vi "Chrg_Dschrg.vi"() -> ()   [LabVIEW 2020]
uses:
  <instrlib>/NH Research Regenerative Test Series/Public/Data/Read (Ave Current).vi
  <instrlib>/NH Research Regenerative Test Series/Public/Data/Low Level/Fetch (Ave Voltage).vi
  <instrlib>/NH Research Regenerative Test Series/NH Research Regenerative Test Series.lvlib
  <instrlib>/IT-M3400/IT-M3400.lvlib
panel:
  in  "Battery Type":enum16{"30Q", "40T"}(ring)
  in  "PS type":enum16{"NHR", "ITECH"}(ring)
  in  "#DAQ outputs (1-13)":i32
  out "Read Ave Current (A)":dbl
  out "Read Ave Voltage (V)":dbl
  in  "Charge/discharge":enum8{"Charge", "Discharge"}(ring)
  out "NHR error out":errorcluster
  out "VISA resource name out":refnum<visa-resource-name>
  out "data task error out":errorcluster
  out "data task out":refnum<k21>
  in  "DischargeCyclePath":path=path "C:/Users/ga11/Desktop/VI/results/3PtestCharge.lvm" caption="Filename"
  in  "Data Task in":refnum<k21>
  in  "data task error in":errorcluster
  in  "PS error in":errorcluster caption="NHR error in (no error)"
  in  "PS VISA in":refnum<visa-resource-name>
  in  "Current Setpoint":dbl format="%#.6g"
  in  "Current Cutoff":dbl
  in  "Charge/Discharge Voltage Setpoint":dbl format="%#.6g"
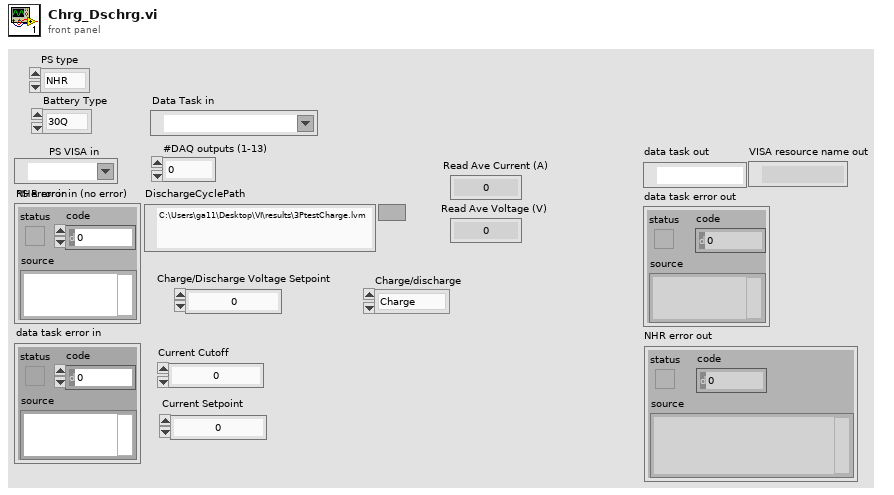
[diagram p1: front panel]
types:
  T1 = cluster{"Voltage Enabled":bool, "Current Enabled":bool, "Power Enabled":bool, "Resistance Enabled":bool}
  T2 = cluster{"Baud Rate":u32, "Parity":u16, "Data Bits":u16, "Stop Bits":u16, "Flow Control":u16}
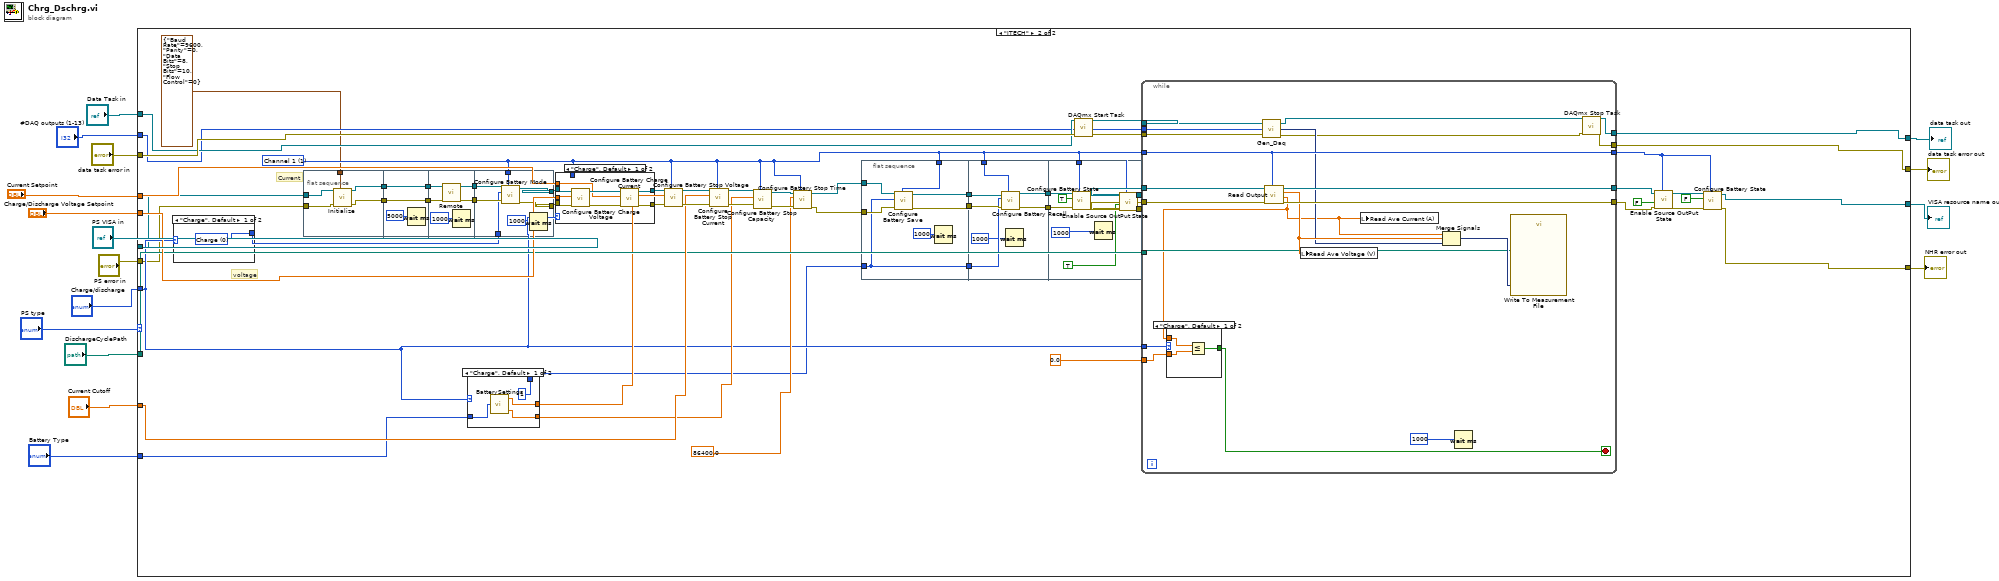
[diagram p0: block diagram]
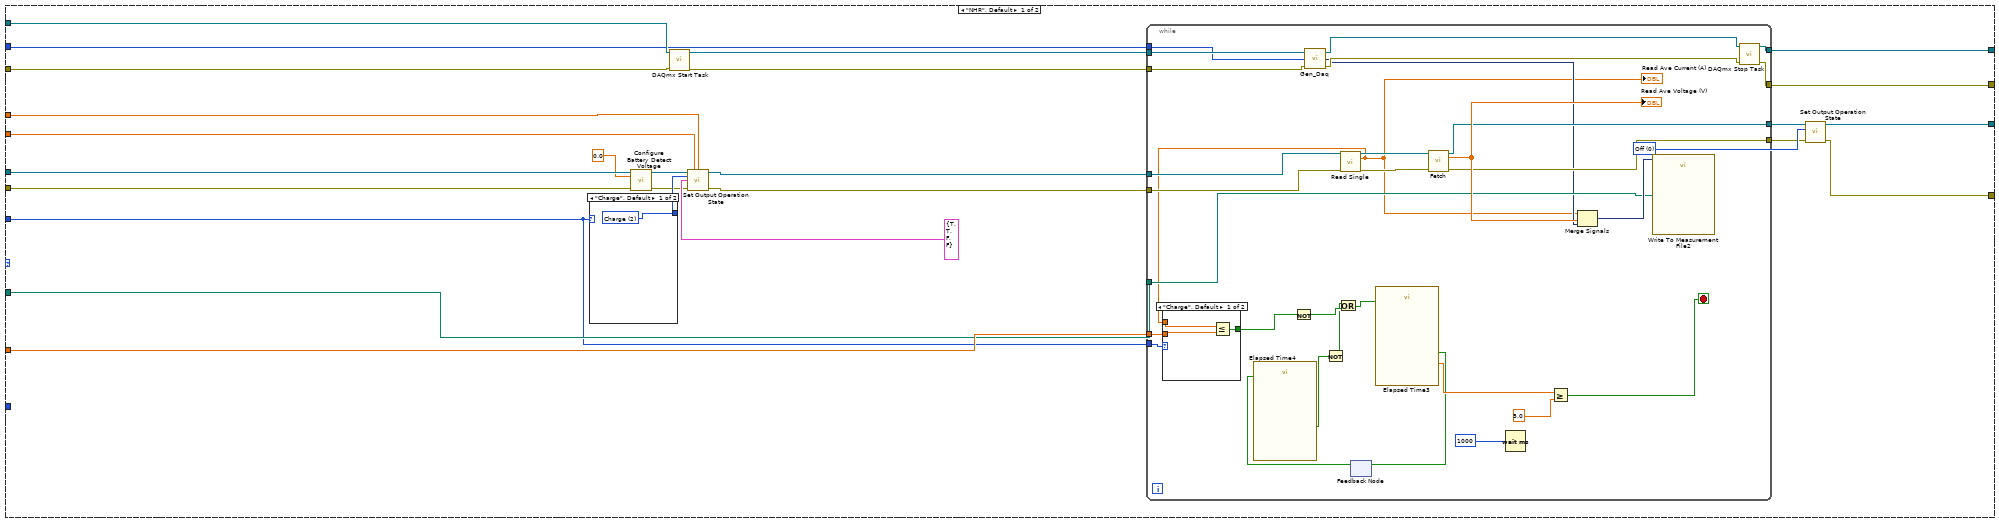
[diagram p2: hidden frame]
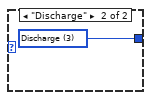
[diagram p3: hidden frame]
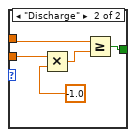
[diagram p4: hidden frame]
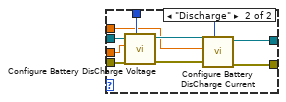
[diagram p5: hidden frame]
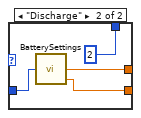
[diagram p6: hidden frame]
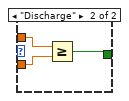
[diagram p7: hidden frame]
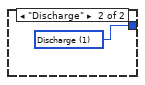
[diagram p8: hidden frame]
diagram:
  n1 = case shown="\"ITECH\"" "PS type" {
    tunnel: "Charge/Discharge Voltage Setpoint" -> [w42 w119]
    tunnel: "Current Setpoint" -> [w17 w112]
    tunnel: "Current Cutoff" -> [w39 w114]
    tunnel: "DischargeCyclePath" -> [w36 w113]
    tunnel: "Data Task in" -> [w33 w120]
    tunnel: "data task error in" -> [w32 w121]
    tunnel: "PS VISA in" -> [w28 w85]
    tunnel: "PS error in" -> [w27 w84]
    tunnel: [w25 w118] -> w8
    tunnel: [w24 w116] -> w7
    tunnel: [w23 w117] -> w6
    tunnel: [w22 w115] -> w5
    tunnel: "Charge/discharge" -> [w18 w106]
    tunnel: "#DAQ outputs (1-13)" -> [w19 w92]
    tunnel: "Battery Type" -> [_ w111]
    frame "NHR", Default {
      w31 = 0 items=["Off", "Standby", "Charge", "Discharge", "Battery"] ("Mode (0: Off)")
      n2 = case shown="\"Charge\", Default" w18 {
        tunnel: [w43 w44] -> w37
        frame "Charge", Default {
          w43 = 2 items=["Off", "Standby", "Charge", "Discharge", "Battery"] ("Mode (0: Off)")
        }
        frame "Discharge" {
          w44 = 3 items=["Off", "Standby", "Charge", "Discharge", "Battery"] ("Mode (0: Off)")
        }
      }
      n3 = call <instrlib>:"Configure Battery Detect Voltage.vi"("VISA resource name"=w28, "Battery Detect Voltage (0V)"=0.0, "error in (no error)"=w27) -> ("VISA resource name out"=w30:refnum<visa-resource-name>, "error out"=w29:errorcluster)  [unwired: 11 in]
      n4 = call <vilib>:"DAQmx Start Task.vi"("task/channels in"=w33, "error in"=w32) -> ("task out"=w35:refnum<k21>, "error out"=w34:errorcluster)  [unwired: 12 in]
      n5 = call <vilib>:"Set Output Operation State.vi"("VISA resource name"=w30, "Voltage Setpoint (0 V)"=w42, "Current Setpoint (0 A)"=w17, "Mode (0: Off)"=w37, "Enable"=T1 {"Voltage Enabled"=TRUE, "Current Enabled"=TRUE, "Power Enabled"=FALSE, "Resistance Enabled"=FALSE}, "error in (no error)"=w29) -> ("VISA resource name out"=w41:refnum<visa-resource-name>, "error out"=w40:errorcluster)  [unwired: 8 in]
      n6 = while {
        tunnel: w41 -> [w73]
        tunnel: w40 -> [w72]
        tunnel: w39 -> [w48]
        tunnel: w34 -> [w53]
        tunnel: w35 -> [w54]
        tunnel: w36 -> [w59]
        tunnel: [w58] -> w25
        tunnel: [w57] -> w23
        tunnel: [w56] -> w21
        tunnel: [w55] -> w20
        tunnel: w19 -> [w52]
        tunnel: w18 -> [w47]
        stop <- w62 stop-if-true
        n7 = call "Gen_Daq.vi"("error in"=w53, "#DAQ outputs (1-13)"=w52, "task/channels in"=w54) -> ("error out"=w50:errorcluster, "DaQ_output"=w49:dynamicdata, "task out"=w51:refnum<k21>)
        n8 = call-poly <instrlib>:"Read Single.vi"("VISA resource name"=w73, "error in (no error)"=w72) -> ("VISA resource name out"=w74:refnum<visa-resource-name>, "Ave Current (A)"=w46:dbl, "error out"=w75:errorcluster)  [unwired: 11 in]
        "Read Ave Current (A)" <- w46
        n9 = case shown="\"Charge\", Default" w47 {
          tunnel: w48 -> [w77 w82]
          tunnel: w46 -> [w78 w80]
          tunnel: [w76 w79] -> w45
          frame "Charge", Default {
            n10 = Less Or Equal?(x=w78, y=w77) -> (x <= y?=w76:bool)
          }
          frame "Discharge" {
            n11 = Multiply(x=w82, y=-1.0) -> (x*y=w81:dbl)
            n12 = Greater Or Equal?(x=w80, y=w81) -> (x >= y?=w79:bool)
          }
        }
        n13 = Not(x=w45) -> (.not. x?=w68:bool)
        n14 = feedback #1() -> (w60:bool)  [unwired: 1 in]
        n15 = call "Elapsed Time4"("Reset"=w60) -> ("Time has Elapsed"=w67:bool)  [unwired: 11 in, 7 out]
        n16 = Not(x=w67) -> (.not. x?=w66:bool)
        n17 = Or(x=w66, y=w68) -> (x .or. y?=w65:bool)
        n18 = call "Elapsed Time3"("Reset"=w65) -> ("Elapsed Time (s)"=w64:dbl, "Time has Elapsed"=w61:bool)  [unwired: 11 in, 6 out]
        n19 = feedback-in #1(w61) -> ()
        n20 = call-poly <instrlib>:"Fetch.vi"("VISA resource name"=w74, "error in (no error)"=w75) -> ("VISA resource name out"=w56:refnum<visa-resource-name>, "Ave Voltage (V)"=w70:dbl, "error out"=w55:errorcluster)  [unwired: 11 in]
        "Read Ave Voltage (V)" <- w70
        n21 = Wait (ms)(milliseconds to wait=1000) -> ()  [unwired: 1 out]
        n22 = Greater Or Equal?(x=w64, y=5.0) -> (x >= y?=w62:bool)
        n23 = Merge Signals "Merge Signals"(w46, w70, w49) -> (w71:dynamicdata)
        n24 = call "Write To Measurement File2"("Signals"=w71, "Filename"=w59) -> ()  [unwired: 15 in, 3 out]
        n25 = call <vilib>:"DAQmx Stop Task.vi"("task/channels in"=w51, "error in"=w50) -> ("task out"=w58:refnum<k21>, "error out"=w57:errorcluster)  [unwired: 12 in]
      }
      n26 = call <vilib>:"Set Output Operation State.vi"("VISA resource name"=w21, "Mode (0: Off)"=w31, "error in (no error)"=w20) -> ("VISA resource name out"=w24:refnum<visa-resource-name>, "error out"=w22:errorcluster)  [unwired: 11 in]
    }
    frame "ITECH" {
      w91 = 1 items=["Channel 1"=1, "Channel 2"=2, "Channel 3"=3, "Channel 4"=4, "Channel 5"=5, "Channel 6"=6, "Channel 7"=7, "Channel 8"=8, "Channel 8"=9, "Channel 10"=10, "Channel 11"=11, "Channel 12"=12, "Channel 13"=13, "Channel 14"=14, "Channel 15"=15, "Channel 16"=16] ("Channel")
      # "voltage"
      # "Current"
      n27 = case shown="\"Charge\", Default" w106 {
        tunnel: [w237 w238] -> w95
        frame "Charge", Default {
          w237 = u8 0 items=["Charge", "Discharge"] ("Battery Mode")
        }
        frame "Discharge" {
          w238 = u8 1 items=["Charge", "Discharge"] ("Battery Mode")
        }
      }
      n28 = flat-sequence {
        tunnel: [w141] -> w89
        tunnel: [w142] -> w87
        tunnel: T2 {"Baud Rate"=9600, "Parity"=0, "Data Bits"=8, "Stop Bits"=10, "Flow Control"=0} ("Serial Configuration") -> [w145]
        tunnel: w84 -> [w144]
        tunnel: w85 -> [w143]
        tunnel: w89 -> [w148]
        tunnel: [w148] -> w88
        tunnel: w87 -> [w147]
        tunnel: [w147] -> w86
        tunnel: [w153] -> w97
        tunnel: [w152] -> w96
        tunnel: w88 -> [w151]
        tunnel: w86 -> [w150]
        tunnel: w97 -> [w157]
        tunnel: w96 -> [w159]
        tunnel: w91 -> [w160]
        tunnel: w95 -> [w158]
        tunnel: [w156] -> w94
        tunnel: [w155] -> w93
        frame #0 {
          n29 = call <instrlib>:"Initialize.vi"("Serial Configuration"=w145, "error in"=w144, "VISA resource name"=w143) -> ("error out"=w142:errorcluster, "VISA resource name out"=w141:refnum<visa-resource-name>)  [unwired: 7 in]
        }
        frame #1 {
          n30 = Wait (ms)(milliseconds to wait=5000) -> ()  [unwired: 1 out]
        }
        frame #2 {
          n31 = call <instrlib>:"Remote.vi"("error in"=w150, "VISA resource name"=w151) -> ("error out"=w152:errorcluster, "VISA resource name out"=w153:refnum<visa-resource-name>)  [unwired: 8 in]
          n32 = Wait (ms)(milliseconds to wait=1000) -> ()  [unwired: 1 out]
        }
        frame #3 {
          n33 = call <instrlib>:"Configure Battery Mode.vi"("Channel"=w160, "error in"=w159, "Battery Mode"=w158, "VISA resource name"=w157) -> ("error out"=w156:errorcluster, "VISA resource name out"=w155:refnum<visa-resource-name>)  [unwired: 6 in]
          n34 = Wait (ms)(milliseconds to wait=1000) -> ()  [unwired: 1 out]
        }
      }
      n35 = case shown="\"Charge\", Default" w106 {
        tunnel: w111 -> [w205 w209]
        tunnel: [w204 w208] -> w110
        tunnel: [w203 w207] -> w109
        tunnel: [u8 1 ("File") u8 2 ("File")] -> w103
        frame "Charge", Default {
          n36 = call "BatterySettings.vi"("Battery Type"=w205) -> ("RatedCapacity (Ah)"=w203:dbl, "Max Voltage (V)"=w204:dbl)  [unwired: 2 in, 1 out]
        }
        frame "Discharge" {
          n37 = call "BatterySettings.vi"("Battery Type"=w209) -> ("RatedCapacity (Ah)"=w207:dbl, "Min Voltage (V)"=w208:dbl)  [unwired: 2 in, 1 out]
        }
      }
      n38 = case shown="\"Charge\", Default" w106 {
        tunnel: w93 -> [w192 w201]
        tunnel: w94 -> [w191 w200]
        tunnel: [w186 w197] -> w130
        tunnel: [w185 w196] -> w129
        tunnel: w91 -> [_ w195]
        tunnel: w119 -> [w188 w194]
        tunnel: w112 -> [w187 w193]
        frame "Charge", Default {
          n39 = call <instrlib>:"Configure Battery Charge Voltage.vi"("error in"=w191, "Charge Voltage(V)"=w188, "VISA resource name"=w192) -> ("error out"=w189:errorcluster, "VISA resource name out"=w190:refnum<visa-resource-name>)  [unwired: 6 in]
          n40 = call <instrlib>:"Configure Battery Charge Current.vi"("error in"=w189, "Charge Current(A)"=w187, "VISA resource name"=w190) -> ("error out"=w185:errorcluster, "VISA resource name out"=w186:refnum<visa-resource-name>)  [unwired: 7 in]
        }
        frame "Discharge" {
          n41 = call <instrlib>:"Configure Battery DisCharge Voltage.vi"("Channel"=w195, "error in"=w200, "Discharge Voltage(V)"=w194, "VISA resource name"=w201) -> ("error out"=w198:errorcluster, "VISA resource name out"=w199:refnum<visa-resource-name>)  [unwired: 6 in]
          n42 = call <instrlib>:"Configure Battery DisCharge Current.vi"("Channel"=w195, "error in"=w198, "Discharge Current(A)"=w193, "VISA resource name"=w199) -> ("error out"=w196:errorcluster, "VISA resource name out"=w197:refnum<visa-resource-name>)  [unwired: 6 in]
        }
      }
      n43 = call <instrlib>:"Configure Battery Stop Voltage.vi"("Channel"=w91, "error in"=w129, "Stop Voltage(V)"=w110, "VISA resource name"=w130) -> ("error out"=w139:errorcluster, "VISA resource name out"=w140:refnum<visa-resource-name>)  [unwired: 6 in]
      n44 = call <instrlib>:"Configure Battery Stop Current.vi"("Channel"=w91, "error in"=w139, "Stop Current(A)"=w114, "VISA resource name"=w140) -> ("error out"=w137:errorcluster, "VISA resource name out"=w138:refnum<visa-resource-name>)  [unwired: 6 in]
      n45 = call <instrlib>:"Configure Battery Stop Capacity.vi"("Channel"=w91, "error in"=w137, "Stop Capacity(Ah)"=w109, "VISA resource name"=w138) -> ("error out"=w135:errorcluster, "VISA resource name out"=w136:refnum<visa-resource-name>)  [unwired: 6 in]
      n46 = call <instrlib>:"Configure Battery Stop Time.vi"("Channel"=w91, "error in"=w135, "Stop Time(S)"=86400.0, "VISA resource name"=w136) -> ("error out"=w99:errorcluster, "VISA resource name out"=w98:refnum<visa-resource-name>)  [unwired: 6 in]
      n47 = flat-sequence {
        tunnel: w103 -> [w166]
        tunnel: w91 -> [w161]
        tunnel: [w164] -> w102
        tunnel: [w166] -> w101
        tunnel: [w163] -> w100
        tunnel: w99 -> [w167]
        tunnel: w98 -> [w165]
        tunnel: [w170] -> w105
        tunnel: [w171] -> w104
        tunnel: w102 -> [w174]
        tunnel: w101 -> [w173]
        tunnel: w100 -> [w172]
        tunnel: w91 -> [w168]
        tunnel: [w178] -> w128
        tunnel: [w177] -> w127
        tunnel: w91 -> [w176]
        tunnel: w105 -> [w184]
        tunnel: w104 -> [w183]
        frame #0 {
          n48 = call <instrlib>:"Configure Battery Save.vi"("Channel"=w161, "error in"=w167, "File"=w166, "VISA resource name"=w165) -> ("error out"=w164:errorcluster, "VISA resource name out"=w163:refnum<visa-resource-name>)  [unwired: 6 in]
          n49 = Wait (ms)(milliseconds to wait=1000) -> ()  [unwired: 1 out]
        }
        frame #1 {
          n50 = call <instrlib>:"Configure Battery Recall.vi"("Channel"=w168, "error in"=w174, "File"=w173, "VISA resource name"=w172) -> ("error out"=w171:errorcluster, "VISA resource name out"=w170:refnum<visa-resource-name>)  [unwired: 6 in]
          n51 = Wait (ms)(milliseconds to wait=1000) -> ()  [unwired: 1 out]
        }
        frame #2 {
          n52 = call <instrlib>:"Configure Battery State.vi"("Channel"=w176, "error in"=w183, "State"=TRUE, "VISA resource name"=w184) -> ("error out"=w181:errorcluster, "VISA resource name out"=w182:refnum<visa-resource-name>)  [unwired: 6 in]
          n53 = Wait (ms)(milliseconds to wait=1000) -> ()  [unwired: 1 out]
          n54 = call <instrlib>:"Enable Source OutPut State.vi"("Channel"=w176, "error in"=w181, "State"=TRUE ("Enable Output|Intput"), "VISA resource name"=w182) -> ("error out"=w177:errorcluster, "VISA resource name out"=w178:refnum<visa-resource-name>)  [unwired: 6 in]
        }
      }
      n55 = call <vilib>:"DAQmx Start Task.vi"("task/channels in"=w120, "error in"=w121) -> ("task out"=w123:refnum<k21>, "error out"=w122:errorcluster)  [unwired: 12 in]
      n56 = while {
        tunnel: [w230] -> w126
        tunnel: [w229] -> w125
        tunnel: w128 -> [w228]
        tunnel: w127 -> [w227]
        tunnel: w91 -> [w226]
        tunnel: [w226] -> w124
        tunnel: w123 -> [w223]
        tunnel: w122 -> [w222]
        tunnel: w92 -> [w219]
        tunnel: [w218] -> w118
        tunnel: [w217] -> w117
        tunnel: w113 -> [w215]
        tunnel: 0.0 -> [w213]
        tunnel: w106 -> [w210]
        stop <- w211 stop-if-true
        n57 = call "Gen_Daq.vi"("error in"=w222, "#DAQ outputs (1-13)"=w219, "task/channels in"=w223) -> ("error out"=w220:errorcluster, "DaQ_output"=w224:dynamicdata, "task out"=w221:refnum<k21>)
        n58 = call <instrlib>:"Read Output.vi"("Channel"=w226, "error in"=w227, "VISA resource name"=w228) -> ("error out"=w229:errorcluster, "Read Current(A)"=w212:dbl, "Read Voltage(V)"=w225:dbl, "VISA resource name out"=w230:refnum<visa-resource-name>)  [unwired: 5 in]
        n59 = case shown="\"Charge\", Default" w210 {
          tunnel: w213 -> [w232 w235]
          tunnel: w212 -> [w233 w236]
          tunnel: [w231 w234] -> w211
          frame "Charge", Default {
            n60 = Less Or Equal?(x=w233, y=w232) -> (x <= y?=w231:bool)
          }
          frame "Discharge" {
            n61 = Greater Or Equal?(x=w236, y=w235) -> (x >= y?=w234:bool)
          }
        }
        n62 = local write "Read Ave Voltage (V)"(w225) -> ()
        n63 = local write "Read Ave Current (A)"(w212) -> ()
        n64 = Merge Signals "Merge Signals"(w212, w225, w224) -> (w216:dynamicdata)
        n65 = Wait (ms)(milliseconds to wait=1000) -> ()  [unwired: 1 out]
        n66 = call "Write To Measurement File"("Signals"=w216, "Filename"=w215) -> ()  [unwired: 15 in, 3 out]
        n67 = call <vilib>:"DAQmx Stop Task.vi"("task/channels in"=w221, "error in"=w220) -> ("task out"=w218:refnum<k21>, "error out"=w217:errorcluster)  [unwired: 12 in]
      }
      n68 = call <instrlib>:"Enable Source OutPut State.vi"("Channel"=w124, "error in"=w125, "State"=FALSE, "VISA resource name"=w126) -> ("error out"=w133:errorcluster, "VISA resource name out"=w134:refnum<visa-resource-name>)  [unwired: 6 in]
      n69 = call <instrlib>:"Configure Battery State.vi"("Channel"=w124, "error in"=w133, "State"=FALSE, "VISA resource name"=w134) -> ("error out"=w115:errorcluster, "VISA resource name out"=w116:refnum<visa-resource-name>)  [unwired: 6 in]
    }
  }
  "data task out" <- w8
  "VISA resource name out" <- w7
  "data task error out" <- w6
  "NHR error out" <- w5
